vi "Get Next Event 1.1.vi"(9 "Exit Event":string, 11 "event queue in":string[](array[string])) -> (0 "Condition (Exit:F)":bool, 2 "next event":string, 3 "event queue out":string[](array[string]), 5 "Previous Event":string)   [LabVIEW 2018]
doc: "Example of implementing an architecture for interactive LabVIEW applications. See the \"Interactive Architectures Revisited\" article in the LabVIEW Technical Resource newsletter, Spring 1996 issue for more details.\n\nSubscribe to the LabVIEW Technical Resource newsletter!\nContact:\nLTR Publishing\n5614 Anita\nDallas, TX 75206\n(214) 827-9931\nFAX (214) 827-9932\nemail ltrsub@aol.com"
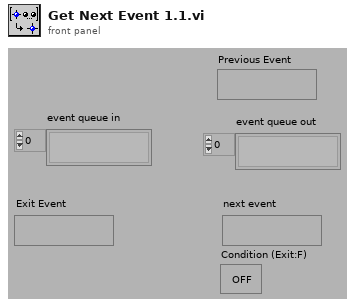
[diagram p1: front panel]
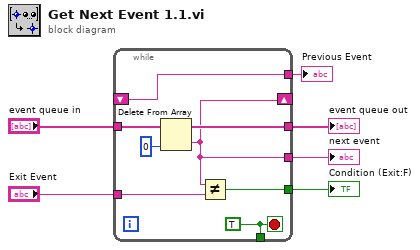
[diagram p0: block diagram]
diagram:
  n1 = while {
    tunnel: [w14] -> w6
    tunnel: "event queue in" -> [w13]
    tunnel: [w11] -> w4
    tunnel: "Exit Event" -> [w10]
    tunnel: [w9] -> w2
    shift-right: [w9] -> _
    shift-left: _ -> [w8]
    tunnel: [w8] -> w1
    tunnel: [w7] -> _
    stop <- w7 stop-if-true
    w7 = TRUE
    n2 = Delete From Array(array=w13, index=0 ("Index")) -> (deleted portion=w9:string, array with subset deleted=w11:string[])  [unwired: 1 in]
    n3 = Not Equal?(x=w9, y=w10) -> (x != y?=w14:bool)
  }
  "event queue out" <- w4
  "next event" <- w2
  "Condition (Exit:F)" <- w6
  "Previous Event" <- w1
